vi "Teleop.vi"(10 "Match Info":T1={"Autonomous Elapsed Seconds"=0.0, "TeleOp Elapsed Seconds"=0.0, "Disabled Elapsed Seconds"=0.0, "Visited Autonomous"=FALSE, "Visited TeleOp"=FALSE, "Visited Disabled"=FALSE, "Autonomous Settings"={"Autonomous Style"=enum."Independent", "VI Refnum"=refnum}}, 11 "Call Context":T2) -> ()   [LabVIEW 2013]
doc: "This VI is called for each TeleOp packet received from the DS where the robot is not disabled. It is often used to read from the joysticks and update I/O or to update setpoints for timed control loops. It should complete and return within 20 milliseconds or it may miss DS packets."
uses:
  Robot Global Data.vi
  <vilib>/Rock Robotics/Network Tables/SD Read Number.vi
  <vilib>/Rock Robotics/WPI/DriverStation/WPI_DriverStationMatch Info.ctl
  <vilib>/Rock Robotics/WPI/DriverStation/WPI_DriverStationDerivedRobotMode.ctl
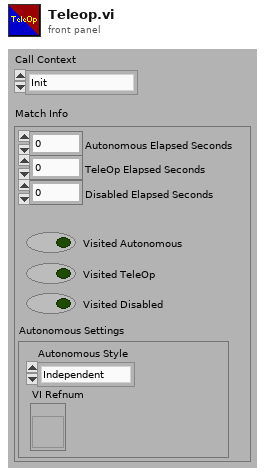
[diagram p1: front panel]
types:
  T1 = typedef "WPI_DriverStationMatch Info.ctl" = cluster{"Autonomous Elapsed Seconds":dbl, "TeleOp Elapsed Seconds":dbl, "Disabled Elapsed Seconds":dbl, "Visited Autonomous":bool, "Visited TeleOp":bool, "Visited Disabled":bool, "Autonomous Settings":cluster{"Autonomous Style":enum16{"Iterative", "Independent"}, "VI Refnum":refnum<vi>}}
  T2 = typedef "WPI_DriverStationDerivedRobotMode.ctl" = enum16{"Init", "Execute", "Stop"}
  T3 = typedef "WPI_JoystickButtonState.ctl" = cluster{"Button 1":bool, "Button 2":bool, "Button 3":bool, "Button 4":bool, "Button 5":bool, "Button 6":bool, "Button 7":bool, "Button 8":bool, "Button 9":bool, "Button 10":bool, "Button 11":bool, "Button 12":bool}
  T4 = cluster{"Axes":cluster{"Joystick 1":cluster{"X Axis":dbl, "Y Axis":dbl}, "Triggers":dbl, "Joystick 2":cluster{"X Axis":dbl, "Y Axis":dbl}}, "Buttons":T3}
  T5 = cluster{"Axes":cluster{"X Axis":dbl, "Y Axis":dbl, "Throttle":dbl, "Unused":dbl, "Unused":dbl, "Unused":dbl}, "Buttons":T3}
  T6 = cluster{"Axes":cluster{"X Axis":dbl, "Y Axis":dbl, "Twist-Handle":dbl, "Throttle":dbl, "Unused":dbl, "Unused":dbl}, "Buttons":T3}
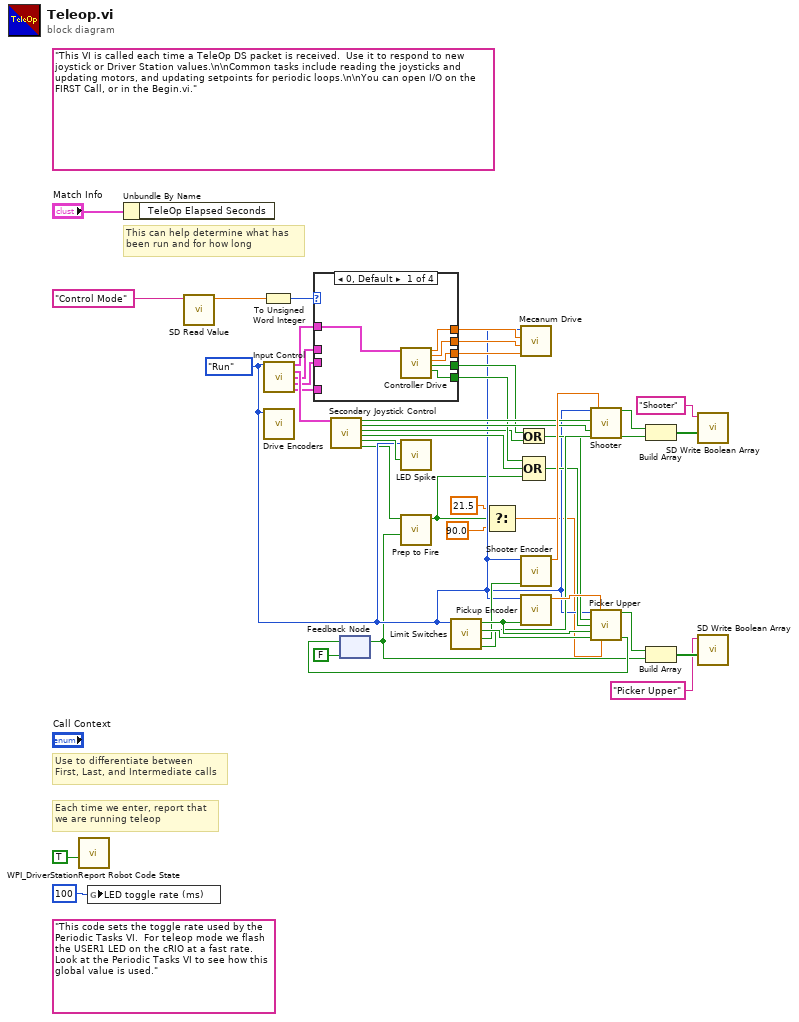
[diagram p0: block diagram]
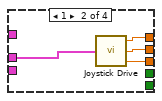
[diagram p2: hidden frame]
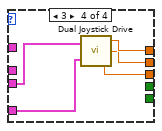
[diagram p4: hidden frame]
diagram:
  w13 = enum16{"Open", "Run", "End"}."Run" ("State")
  (unwired) "This code sets the toggle rate used by the Periodic Tasks VI.  For teleop mode we flash the USER1 LED on the cRIO at a fast rate.  Look at the Periodic Tasks VI to see how this global value is used."
  (unwired) "This VI is called each time a TeleOp DS packet is received.  Use it to respond to new joystick or Driver Station values.\n\nCommon tasks include reading the joysticks and updating motors, and updating setpoints for periodic loops.\n\nYou can open I/O on the FIRST Call, or in the Begin.vi."
  # "Each time we enter, report that\nwe are running teleop"
  # "Use to differentiate between\nFirst, Last, and Intermediate calls"
  # "This can help determine what has\nbeen run and for how long"
  n1 = call <vilib>:"WPI_DriverStationReport Robot Code State.vi"("TeleOp"=TRUE ("Autonomous")) -> ()  [unwired: 10 in, 1 out]
  n2 = global write "Robot Global Data.vi" "LED toggle rate (ms)"(u32 100 ("LED ms toggle rate")) -> ()
  n3 = Unbundle By Name("Match Info") -> ()  [unwired: 1 out]
  n4 = call-poly <vilib>:"SD Read Value.vi"("Name"="Control Mode") -> ("Numeric"=w41:dbl)  [unwired: 8 in, 2 out]
  n5 = To Unsigned Word Integer(number=w41) -> (unsigned 16bit integer=w40:u16)
  n6 = call "Input Control.vi"("State"=w13) -> ("Gamepad"=w39:T4, "Secondary Joystick"=w29:T5, "Twist-handle Joystick"=w3:T6, "Dual Joystick 1"=w2:T5, "Dual Joystick 2"=w1:T5)  [unwired: 10 in]
  n7 = call "Drive Encoders.vi"("State Control"=w13) -> ()  [unwired: 3 in, 4 out]
  n8 = case shown="0, Default" w40 {
    tunnel: w39 -> [w51 _ _ _]
    tunnel: [w50 w54 _ w60] -> w38
    tunnel: [w49 w53 _ w59] -> w37
    tunnel: [w48 w52 _ w58] -> w36
    tunnel: [w47 _ _ _] -> w21
    tunnel: [w46 _ _ _] -> w24
    tunnel: w3 -> [_ w55 _ _]
    tunnel: w2 -> [_ _ _ w57]
    tunnel: w1 -> [_ _ _ w56]
    frame 0, Default {
      n9 = call "Controller Drive.vi"("input cluster"=w51) -> ("Strafe"=w50:dbl, "Forward/Reverse"=w49:dbl, "Turn"=w48:dbl, "Picker Upper Up"=w47:bool, "Picker Upper Down"=w46:bool)  [unwired: 14 in]
    }
    frame 1 {
      n10 = call "Joystick Drive.vi"("Joystick Drive"=w55) -> ("Strafe"=w54:dbl, "Forward/Backward"=w53:dbl, "Turn"=w52:dbl)
    }
    frame 2 {
    }
    frame 3 {
      n11 = call "Dual Joystick Drive.vi"("Joystick 1"=w57, "Joystick 2"=w56) -> ("Strafe"=w60:dbl, "Forward/Backward"=w59:dbl, "Turn"=w58:dbl)
    }
  }
  n12 = call "Secondary Joystick Control.vi"("Secondary Joystick"=w29) -> ("Shooter return"=w28:bool, "Shooter 4 feet"=w27:bool, "Picker upper up"=w22:bool, "Picker upper down"=w25:bool, "LED"=w26:bool, "Fire\nPreset"=w12:bool)  [unwired: 13 in]
  n13 = feedback #1(FALSE ("Fully down?")) -> (w10:bool)
  n14 = call "LED Spike.vi"("ON/OFF"=w26, "State"=w13) -> ()  [unwired: 10 in]
  n15 = call "Prep to Fire.vi"("Fully down?"=w10, "Input"=w12) -> ("Latched"=w8:bool)  [unwired: 9 in]
  n16 = call "Limit Switches.vi"("State Control"=w13) -> ("Shooter Top"=w30:bool, "Shooter Bottom"=w32:bool, "Picker Upper Bottom"=w33:bool, "Picker Upper Top"=w34:bool)  [unwired: 7 in]
  n17 = Select(t=21.5, s=w8, f=90.0) -> (s? t:f=w5:dbl)
  n18 = Or(x=w21, y=w22) -> (x .or. y?=w20:bool)
  n19 = call "Mecanum Drive.vi"("Turn"=w36, "Forward/Backward"=w37, "Strafe"=w38, "State Control"=w13) -> ()  [unwired: 4 in]
  n20 = call "Shooter Encoder.vi"("Reset Encoder?"=w32, "State Control"=w13) -> ("Encoder Degrees"=w31:dbl)  [unwired: 2 in, 3 out]
  n21 = call "Pickup Encoder.vi"("Reset Encoder?"=w34, "State Control"=w13) -> ("Encoder Degrees"=w35:dbl)  [unwired: 2 in, 3 out]
  n22 = Compound Arithmetic op=OR(w24, w25, w8) -> (w23:bool)
  n23 = call "Shooter.vi"("State Control"=w13, "Return"=w28, "4 ft"=w27, "Top Limit"=w30, "Encoder"=w31) -> ("Fully shot?"=w19:bool, "Fully retracted?"=w18:bool)  [unwired: 13 in]
  n24 = call "Picker Upper.vi"("State Control"=w13, "Encoder"=w35, "Up"=w20, "Down"=w23, "Top limit"=w34, "Bottom Limit"=w33, "Down break"=w5) -> ("Fully up?"=w4:bool, "Fully down?"=w11:bool)  [unwired: 7 in]
  n25 = feedback-in #1(w11) -> ()
  n26 = Build Array(w19, w18) -> (w17:bool[])
  n27 = Build Array(w4, w10) -> (w15:bool[])
  n28 = call <vilib>:"SD Write Boolean Array.vi"("Boolean Array"=w17, "Name"="Shooter") -> ()  [unwired: 8 in, 2 out]
  n29 = call <vilib>:"SD Write Boolean Array.vi"("Boolean Array"=w15, "Name"="Picker Upper") -> ()  [unwired: 8 in, 2 out]
